vi "Exemple_Preprocessing_add_dummy_feature.vi"() -> ()   [LabVIEW 2020]
panel:
  in  "Type X":enum16{"Array", "Sparse"}(ring)
  out "Data":T1
  out "error out":errorcluster
  in  "X":string[][](array[string])=[["0", "1"], ["1", "0"]]
  in  "error in":errorcluster caption="entrée d'erreur"
  in  "add_dummy_feature":cluster{"value":dbl}={"value"=1.0}
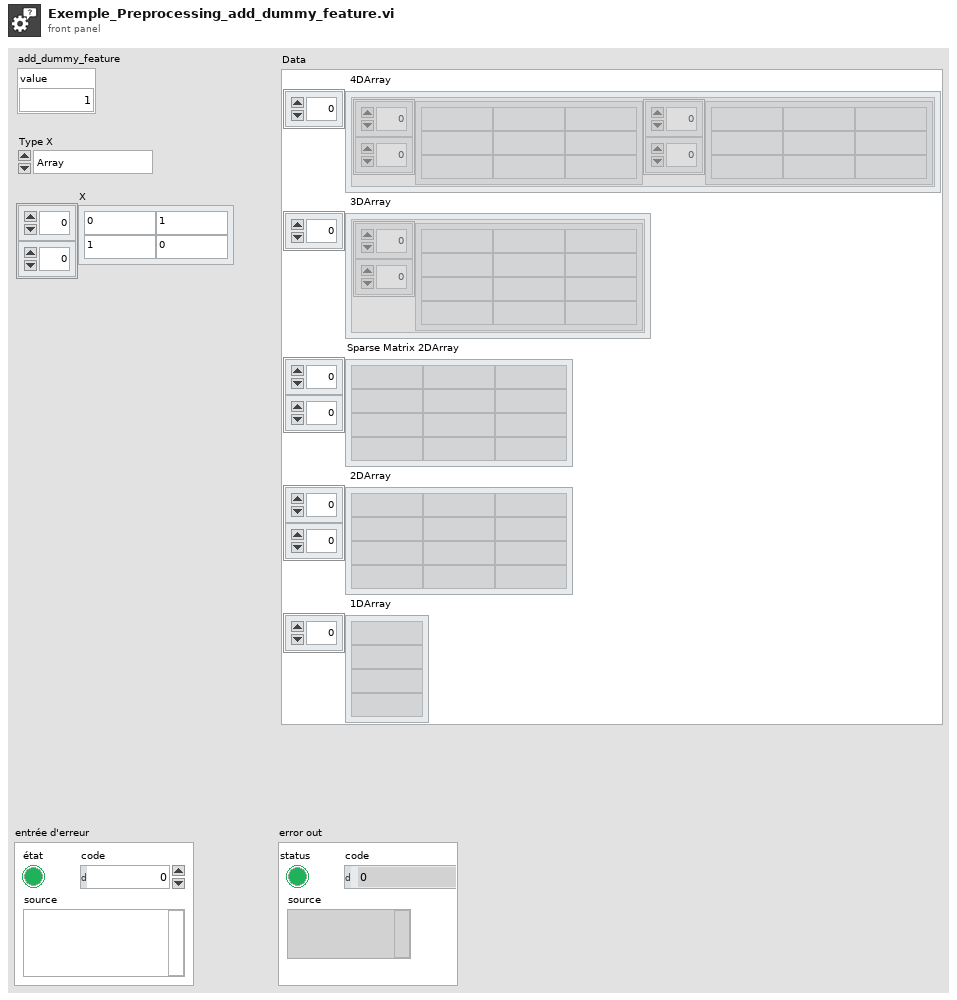
[diagram p1: front panel]
types:
  T1 = cluster{" 4DArray":cluster{"1":string[][], "2":string[][]}[], " 3DArray":cluster{"Tableau":string[][]}[], "Sparse Matrix 2DArray":string[][], " 2DArray":string[][], " 1DArray":string[]}
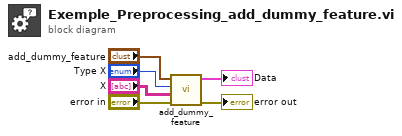
[diagram p0: block diagram]
diagram:
  n1 = call "add_dummy_feature.vi"("error in"="error in", "X"="X", "Type X"="Type X", "add_dummy_feature"="add_dummy_feature") -> ("error out"=→"error out":errorcluster, "Data"=→"Data":T1)  [unwired: 6 in]
